vi "focusvi.vi"(1 "zc":dbl=5.0, 2 "yc":dbl, 3 "xc":dbl) -> (0 "finalz":dbl)   [LabVIEW 2015]
uses:
  <vilib>/Utility/miscctls.llb/LVOffsetAndMultiplierTypeDef.ctl
  <vilib>/DAQmx/read.llb/DAQmx Read (Analog 2D I16 NChan NSamp).vi
  <vilib>/DAQmx/write.llb/DAQmx Write (Analog DBL 1Chan 1Samp).vi
  Misc/add channel to active arrayv2.vi
  <vilib>/DAQmx/miscellaneous.llb/DAQmx Fill In Error Info.vi
  <vilib>/DAQmx/create/channels.llb/DAQmx Create Channel (AO-Voltage-Basic).vi
panel:
  in  "objective":u16(ring) items=["Olympus 25x NA 1.05", "Olympus 60x NA 1.2"]
  out "zsteps":i16
  out "ysteps":i16
  out "xsteps":i16
  out "samples":i32=18000
  in  "stop":bool
  in  "z-":bool
  in  "z+":bool
  in  "y+":bool
  in  "y-":bool
  in  "x+":bool
  in  "x-":bool
  in  "stepsize":dbl=0.005
  in  "zamp":dbl=0.25
  in  "y amp":dbl=0.25
  in  "x amp":dbl=0.25
  in  "samplingrate":dbl=18000.0
  in  "frametime (s)":dbl=1.0
  out "Waveform Graph 6":dbl[][](graph)=[[-0.004837577472790145, -0.005916214699391275, -0.005143459723331034, -0.0050629642879357565, -0.0055942334933206436, -0.004934171959757805, -0.004869775637052954, -0.005900115636177361, -0.004837577484431676, -0.005272252205759287, -0.00519175692461431, -0.005175657814834267, -0.004918072849977762, -0.005594233502051793, -0.0048214784445008265, -0.004563893371960148, -0.005191756977001205, -0.006286493106745184, -0.006318691279739141, -0.006431384710595012, -0.0047409831633558495, -0.00449949721514713, -0.005095162519137375, -0.005706926877610386, -0.005449341842904687, -0.004274110283586196, -0.004258011243655347, -0.00601280911359936, -0.005159558818559162, -0.004467299010138958, -0.005658629696699791, -0.005401044723112136, -0.0056425306131131945, -0.005465440975967795, -0.005030766304116696, -0.004499497218057513, -0.0048858746944461014, -0.004998568107839674, -0.005079063423909247, -0.005996709992177785, -0.004628289659740404, -0.0061416015611030165, -0.004531695364858024, -0.0050146671332186084, -0.005803521323832684, -0.005803521280176938, -0.004419001890346408, -0.005288351277704351, -0.0052078558917855846, -0.004354605649132282, -0.0052400540531380106, -0.004918072823784314, -0.006238195998594165, -0.004918072803411633, -0.004531695260084234, -0.006592375377658754, -0.005384945645346306, -0.003919930930715054, -0.003098878636956215, -0.005240054079331457, -0.0050790634355507795, -0.005223955085966736, -0.005513738165609539, -0.005578134371899068, -0.005417143856175244, -0.005143459711689502, -0.004274110251571983, -0.005352747463621199, -0.006705068866722286, -0.004402902800939046, -0.005626431608106941, -0.004982469088281505, -0.004934171901550144, -0.00588401664281264, -0.005368846619967371, -0.005787422135472298, -0.005143459743703715, -0.005449341842904687, -0.005884016584604979, -0.005626431573182345, -0.005513738165609539, -0.005690827895887196, -0.005449341936036944, -0.005497638962697238, -0.006205997802317143, -0.0052400540531380106, -0.004386803656234406, -0.00507906349375844, -0.005079063517041504, -0.005916214757598936, -0.005079063412267715, -0.0057391250040382145, -0.005916214716853574, -0.005143459673854522, -0.005755224090535194, -0.005610332533251494, -0.004354605588014237, -0.005417143751401454, -0.005384945636615157, -0.005352747425786219], [-0.004950270894914866, -0.005529837135691195, -0.004740983113879338, -0.004080921574495733, -0.0051595588098280135, -0.004644388775341212, -0.005175657826475799, -0.004612190602347255, -0.0058035212336108085, -0.005288351303897798, -0.00470878497872036, -0.006286493176594377, -0.0042741102486616, -0.004435100889531895, -0.005835719360038638, -0.00532054939540103, -0.005513738142326474, -0.005207855929620564, -0.003791138363885693, -0.00498246910283342, -0.00522395505104214, -0.0051112615590682255, -0.005401044804602862, -0.004805379404569976, -0.004982469041715376, -0.005159558771993034, -0.005401044629979879, -0.005175657838117331, -0.00546544095268473, -0.005352747399592772, -0.004982469032984227, -0.005143459662212991, -0.005240054125897587, -0.005578134371899068, -0.004934171889908611, -0.005465440987609327, -0.004966369981411844, -0.0050307662691921, -0.0041453178244410084, -0.004757082191645168, -0.005336648505181074, -0.004628289659740404, -0.0058035212336108085, -0.00618989875074476, -0.004740983081865125, -0.004918072800501249, -0.004901973728556186, -0.005159558771993034, -0.005288351280614734, -0.00522395505104214, -0.005674728751182556, -0.004869775645784102, -0.003952129045501351, -0.0045316952717257665, -0.0054171438212506475, -0.005175657791551202, -0.004918072780128568, -0.005240054085152224, -0.005352747533470393, -0.00561033247213345, -0.004934171820059419, -0.0056586296646855775, -0.005320549383759499, -0.005062964372336864, -0.005207855964545161, -0.005384945613332093, -0.00496636992902495, -0.0042902093147858976, -0.0045316953299334274, -0.005336648470256477, -0.004837577464058995, -0.00535274749272503, -0.005062964430544525, -0.005529837228823453, -0.005578134418465197, -0.004612190625630319, -0.006189898820593953, -0.004467299021780491, -0.004869775590486824, -0.00532054940413218, -0.005256153162918054, -0.004708784993272275, -0.004177515907213092, -0.004789280318072997, -0.004966370004694909, -0.005143459723331034, -0.006222096970304847, -0.005433242884464562, -0.005626431608106941, -0.005223954989924095, -0.004113119671819732, -0.004982469126116484, -0.005272252229042351, -0.004805379384197295, -0.004241912145516835, -0.005079063447192311, -0.0051595587545307355, -0.00607720531988889, -0.00578742225188762, -0.004419001864152961]]
  out "Waveform Graph 5":dbl[][](graph)=[[-0.005562035366892815, -0.005562035320326686, -0.005545936292037368, -0.005819620378315449, -0.0056103325448930265, -0.005256153139634989, -0.005384945645346306, -0.004998568102018907, -0.004676586796995253, -0.005288351254421286, -0.005159558821469545, -0.005272252214490436, -0.005771323142107576, -0.005079063400626182, -0.004821478459052742, -0.00429020928859245, -0.0053205494303256275, -0.005465441034175456, -0.005240054044406861, -0.005030766234267503, -0.005336648458614946, -0.004982469126116484, -0.005626431596465409, -0.005095162440557033, -0.005674728751182556, -0.0055137382121756675, -0.005642530621844344, -0.0052239549084333705, -0.00401652529835701, -0.005207855996559374, -0.005851818434894085, -0.0056747287744656205, -0.005384945683181286, -0.005384945633704774, -0.004950270976405591, -0.00524005409097299, -0.005803521230700426, -0.005642530729528516, -0.004628289642278105, -0.004982469091191888, -0.004644388746237382, -0.00541714378632605, -0.005159558742889203, -0.005062964395619929, -0.005352747580036521, -0.005706926932907664, -0.005706926889251918, -0.005578134465031326, -0.005159558786544949, -0.0063830875558778645, -0.004467299015959725, -0.005529837182257325, -0.006189898774027825, -0.00614160159311723, -0.004708785028196871, -0.0054171437659533694, -0.005127360642654821, -0.005449341901112348, -0.004676586936693638, -0.004805379334720783, -0.004789280347176827, -0.005030766254640185, -0.00562643154989928, -0.005578134360257536, -0.0042580112116411325, -0.004998568119481206, -0.005175657800282352, -0.005433242846629582, -0.004338506443309598, -0.0056264315120643, -0.004789280294789933, -0.004097020631888881, -0.005529837205540389, -0.004950270941480994, -0.0054815399926155806, -0.005658629618119448, -0.005079063400626182, -0.005481539922766387, -0.005481540027540177, -0.0055459362803958355, -0.005175657835206948, -0.005288351254421286, -0.005803521303460002, -0.005401044641621411, -0.006173799707903526, -0.005401044720201753, -0.00461219068383798, -0.005851818341761827, -0.004724884033203125, -0.005996710085310042, -0.005014667171053588, -0.005545936338603496, -0.005095162510406226, -0.00581962033174932, -0.004531695286277682, -0.004209713998716324, -0.0037106430681888014, -0.006640672439243644, -0.005690827872604132, -0.005867917533032596], [-0.00441900179721415, -0.00557813432533294, -0.005900115612894297, -0.00470878496998921, -0.005384945645346306, -0.005159558728337288, -0.006012809133972041, -0.0068821584107354285, -0.004740983151714317, -0.005272252194117755, -0.00482147850561887, -0.004370704677421599, -0.005320549383759499, -0.005046865352778695, -0.005578134360257536, -0.005336648420779966, -0.006173799722455442, -0.005851818574592471, -0.004885874659521505, -0.005272252194117755, -0.005706926769926212, -0.006077205296605825, -0.005175657823565416, -0.0045155962376156825, -0.004853676550555974, -0.005658629676327109, -0.0050307662691921, -0.005062964381068014, -0.00495027091819793, -0.004837577504804358, -0.005594233397278004, -0.005272252226131968, -0.005562035320326686, -0.005642530668410473, -0.0050307662226259705, -0.005578134430106729, -0.005240054125897587, -0.005723025975748896, -0.004837577472790145, -0.005111261626007035, -0.004853676570928655, -0.0049663699930533765, -0.006415285679395311, -0.005256153162918054, -0.005272252100985498, -0.006383087439462543, -0.005256153189111501, -0.0051112615590682255, -0.004982469067908823, -0.005207855961634778, -0.004129218746675179, -0.005143459650571458, -0.004676586863934062, -0.00429020939336624, -0.004531695257173851, -0.005095162522047758, -0.006383087509311736, -0.004789280344266444, -0.006061106291599572, -0.005384945729747415, -0.004612190619809553, -0.005352747486904263, -0.004821478453231975, -0.00514345970004797, -0.004596091527491808, -0.005433242802973836, -0.005900115691474639, -0.004547794346581213, -0.006045007181819528, -0.005320549453608691, -0.005240054079331457, -0.006994851885247044, -0.004757082182914018, -0.004435100973933004, -0.005030766280833631, -0.004467299068346619, -0.005111261631827802, -0.00509516254242044, -0.00519175682857167, -0.0050951625453308225, -0.0051112615037709475, -0.005223955027759075, -0.0058679175563156605, -0.004612190599436872, -0.0043385065859183666, -0.006045007123611867, -0.0049824689864180986, -0.005014667205978185, -0.005062964395619929, -0.00486977563414257, -0.004869775648694485, -0.005223954978282564, -0.005111261538695544, -0.004885874700266868, -0.004644388661836274, -0.005739125050604343, -0.005465440871194005, -0.0050951625453308225, -0.004789280297700316, -0.005803521335474215]]
  out "Waveform Graph 4":dbl[][](graph)=[[-0.005288351234048605, -0.0044351008458761495, -0.005417143774684519, -0.005771323153749108, -0.005465441042906605, -0.006061106370179914, -0.004853676515631377, -0.0053205493371933695, -0.005562035366892815, -0.005417143780505285, -0.006045007274951786, -0.005723025952465832, -0.006302592321299016, -0.004676586855202914, -0.005835719406604767, -0.005223955016117543, -0.004209713984164409, -0.0055459363735280934, -0.004805379442404956, -0.004757082171272487, -0.005513738142326474, -0.005175657838117331, -0.0049985682097030805, -0.005062964337412268, -0.0060772053897380825, -0.0053849456220632416, -0.004740983198280447, -0.004869775587576441, -0.005723025984480046, -0.005674728751182556, -0.004869775590486824, -0.005562035297043621, -0.004628289677202702, -0.004644388679298572, -0.0051595587166957555, -0.005111261538695544, -0.004966370036709122, -0.005401044664904475, -0.0060772053897380825, -0.005723025975748896, -0.005433242837898433, -0.005320549372117967, -0.004708784993272275, -0.005095162484212779, -0.004918072870350443, -0.005706926877610386, -0.004901973725645803, -0.004435100883711129, -0.004660487800720148, -0.005288351347553543, -0.005256153177469969, -0.004821478447411209, -0.004708784967078827, -0.005562035366892815, -0.004644388679298572, -0.005658629792742431, -0.004258011269848793, -0.00483757744950708, -0.0048375774989835914, -0.0049019737634807825, -0.004918072823784314, -0.005723025975748896, -0.0056425306713208554, -0.005095162460929714, -0.0051273606484755875, -0.005272252205759287, -0.004724884137976915, -0.006238195998594165, -0.004563893505837769, -0.0054815399926155806, -0.004692685857298784, -0.004354605625849217, -0.005256153113441542, -0.005127360657206736, -0.004869775599217974, -0.005030766266281716, -0.004837577469879761, -0.005207855976186693, -0.005642530624754727, -0.005368846608325839, -0.006431384687311947, -0.005835719371680171, -0.005191756851854734, -0.005304450355470181, -0.005079063444281928, -0.005723025929182768, -0.005272252182476222, -0.004950270915287547, -0.0050146670750109475, -0.005610332611831836, -0.00457999249920249, -0.004885874662431888, -0.005626431581913493, -0.005095162498764694, -0.005674728727899492, -0.004773181278142147, -0.005175657849758863, -0.005964511854108423, -0.005240054032765329, -0.006157700694166124], [-0.005433242849539966, -0.0056747287744656205, -0.005175657916697674, -0.005497639137320221, -0.005771323200315237, -0.00559423347003758, -0.004016525283805095, -0.00517565777990967, -0.005014667203067802, -0.005739124969113618, -0.005433242849539966, -0.004483398119919002, -0.003839435672853142, -0.004805379395838827, -0.004467299018870108, -0.0056908278609626, -0.005884016584604979, -0.00532054939540103, -0.004918072815053165, -0.005014667194336653, -0.004177515939227305, -0.005240054056048393, -0.005256153142545373, -0.0054654409410431985, -0.004934171913191676, -0.005368846585042775, -0.005095162484212779, -0.00538494570646435, -0.004225813108496368, -0.0050468652916606516, -0.0055781344417482615, -0.005159558771993034, -0.005401044664904475, -0.005207855952903628, -0.004515596255077981, -0.005288351257331669, -0.00536884656175971, -0.0049019737838534635, -0.004982469114474952, -0.005932313832454383, -0.004306308436207473, -0.00546544101962354, -0.0055620353319682184, -0.0050146671681432055, -0.005062964372336864, -0.004274110292317346, -0.004789280274417251, -0.005207855848129839, -0.0055459362803958355, -0.005368846535566263, -0.005513738165609539, -0.004402902800939046, -0.004563893331214786, -0.005030766266281716, -0.005803521303460002, -0.00424191213096492, -0.004354605634580367, -0.005256153142545373, -0.004467298983945512, -0.005191756831482053, -0.004467299068346619, -0.005288351234048605, -0.00536884656175971, -0.005175657858490013, -0.0053366483887657525, -0.005352747533470393, -0.0063830874627456066, -0.0049180727772181855, -0.005159558705054223, -0.0050790634355507795, -0.005320549369207584, -0.006833861174527556, -0.00552983716770541, -0.005497639055829495, -0.005449341854546219, -0.004789280306431465, -0.004885874685714953, -0.005916214699391275, -0.004708784958347678, -0.004692685880581848, -0.005642530659679323, -0.005626431584823876, -0.004644388728775084, -0.004821478432859294, -0.005674728684243746, -0.005513738200534135, -0.005658629781100899, -0.006125502567738294, -0.004821478424128145, -0.005223954981192947, -0.005207855952903628, -0.005706926807761192, -0.005240054114256054, -0.005594233423471451, -0.005143459653481841, -0.0054815400508232415, -0.0044029027776559815, -0.0049663699930533765, -0.0052078558946959674, -0.005884016596246511]]
  in  "bin":dbl=20.0
  out "Waveform Graph 3":dbl[][](graph)=[[-0.002712501134374179, -0.002406618936220184, -0.0023100245656678454, -0.0024871142755728214, -0.002245628336095251, -0.00256760960619431, -0.002020241448190063, -0.0024227179790614175, -0.0020202414161758497, -0.002937888045562431, -0.0023261236550752074, -0.0019397461233893409, -0.0022295292728813365, -0.0017787554766982793, -0.0025837086490355433, -0.0023100245569366963, -0.0023744208185235037, -0.0022295292321359737, -0.002310024542384781, -0.0022778264275984837, -0.002116835827473551, -0.0024227179877925665, -0.002213430209667422, -0.002535411441931501, -0.002438817048096098, -0.0022456283215433357, -0.002503213344607502, -0.0021651329938322307, -0.002986185168265365, -0.002020241433638148, -0.002454916134593077, -0.0025676095974631608, -0.0024388170219026505, -0.002664203947642818, -0.0023905198991997167, -0.002004142355872318, -0.0023744208097923546, -0.0026159067871049046, -0.0027929964679060506, -0.002487114261020906, -0.002454916128772311, -0.001875349847250618, -0.0026320058066630738, -0.002132934870314784, -0.0024066189216682687, -0.002342222718289122, -0.0019397461001062766, -0.0025354114535730333, -0.0026320058677811176, -0.0025354114593937995, -0.0021490339480806143, -0.002358321737847291, -0.0026320058357669042, -0.002358321781503037, -0.002454916134593077, -0.002310024536564015, -0.002132934870314784, -0.0025032133125932887, -0.0020846376719418913, -0.0026320057979319243, -0.002197331137722358, -0.0023100245336536316, -0.0021973310853354634, -0.0021329348586732523, -0.0024227179936133327, -0.00232612362888176, -0.002503213335876353, -0.0025032133038621397, -0.002326123652164824, -0.0025354114652145652, -0.002213430171832442, -0.002245628336095251, -0.0023905198933789505, -0.002213430221308954, -0.0020685386116383597, -0.0022778264770749956, -0.0026803030079463495, -0.0023905198991997167, -0.0023905198584543543, -0.0022939254675293343, -0.0025676095683593303, -0.0028734917839756237, -0.0021651329705491664, -0.0024066189245786516, -0.002358321732026525, -0.0024710152094485236, -0.002503213327145204, -0.002760798344388604, -0.002277826436329633, -0.002197331114439294, -0.0025515104876831173, -0.0024388170626480133, -0.0027768973843194543, -0.0020685385970864445, -0.0024871142726624385, -0.0026964020740706473, -0.002792996456264518, -0.0021168358100112526, -0.0022778264275984837, -0.002374420821433887], [-0.0024227180139860137, -0.0023744207981508227, -0.002519312399090268, -0.0023422226775437595, -0.002229529243777506, -0.002567609556717798, -0.0024549160996684806, -0.0022617273643845692, -0.0022134301980258897, -0.0021973311435431243, -0.002213430157280527, -0.002471015212358907, -0.0022939254791708662, -0.002406618944951333, -0.002535411424469203, -0.002310024548205547, -0.0023905198584543543, -0.002116835824563168, -0.002438817039364949, -0.0025515105167869478, -0.0021007367526181043, -0.0025032133009517564, -0.002229529243777506, -0.0027768973930506037, -0.002728600206319243, -0.002471015203627758, -0.001939746068092063, -0.0024066189827863125, -0.002116835824563168, -0.001955845145857893, -0.0023100245656678454, -0.002165133022936061, -0.0027125011867610736, -0.0026481049018912016, -0.0021490339160664005, -0.0027446992986369877, -0.002503213330055587, -0.0025032133155036716, -0.0021651329909218473, -0.002326123625971377, -0.002068538617459126, -0.0023422226717229933, -0.0027607983152847736, -0.0024710151774343103, -0.0022134301863843573, -0.0022134301892947406, -0.0018270526605192571, -0.002744699252070859, -0.0025032133125932887, -0.0026320058037526905, -0.002471015212358907, -0.0021651329851010816, -0.0026320058124838395, -0.0023261236026883127, -0.0025998076889663935, -0.0025837086082901805, -0.0020363404968520627, -0.002664204002940096, -0.002245628274977207, -0.0025354114535730333, -0.0023583217873238025, -0.002068538608727977, -0.0025354114768560976, -0.002277826424688101, -0.0024549161695176735, -0.0021490339393494652, -0.0025515104993246497, -0.002052439551334828, -0.0021007367438869553, -0.0022134301892947406, -0.0023583217291161416, -0.002873491813079454, -0.0020041423529619353, -0.0024227180139860137, -0.002197331137722358, -0.0023100245802197606, -0.0029700861865421756, -0.0024549161025788635, -0.0024549161695176735, -0.0017948545544641092, -0.0027768974483478813, -0.0022617273381911216, -0.0024710151861654594, -0.0027768973930506037, -0.001988043324672617, -0.0024710151978069917, -0.0024388170917518438, -0.002245628341916017, -0.0022617273789364845, -0.0019236470601754264, -0.0026642039709258826, -0.0026320058357669042, -0.0026803030661540104, -0.0024710152443731203, -0.002632005824125372, -0.0023583217611303554, -0.0018914489191956818, -0.0023905198584543543, -0.0021651329938322307, -0.002374420812702738]]
  out "Waveform Graph 2":dbl[][](graph)=[[-0.0022939254879020153, -0.0025676095916423946, -0.002132934902328998, -0.002374420821433887, -0.002390519852633588, -0.002277826436329633, -0.002036340444465168, -0.0026964020653394982, -0.0024388171033933757, -0.0027286002004984766, -0.002374420838896185, -0.002712501146015711, -0.0021812320541357622, -0.002245628318632953, -0.0022939254500670358, -0.0022617273789364845, -0.002583708643214777, -0.002020241413265467, -0.0024710151890758427, -0.002567609547986649, -0.002100736740976572, -0.0024871142988558857, -0.002197331073693931, -0.0025032132922206073, -0.00258370864612516, -0.0021329348644940184, -0.0024710151861654594, -0.002084637639927678, -0.0029861852177418768, -0.0022617273876676335, -0.0025193124020006508, -0.002100736749707721, -0.0024871142813935876, -0.0026481049018912016, -0.002132934870314784, -0.0024388170888414605, -0.002712501198402606, -0.0018592507723951713, -0.0028251945797819642, -0.0022456283011706548, -0.002326123634702526, -0.0022939255024539305, -0.0022456282924395053, -0.002615906766732223, -0.0028734917956171556, -0.002342222651350312, -0.0022295292641501875, -0.0023100245773093773, -0.00255151052842848, -0.002132934870314784, -0.002326123637612909, -0.0019397461146581918, -0.002068538626190275, -0.00263200584158767, -0.00250321333296597, -0.0025837086228420957, -0.001843151735374704, -0.002551510540070012, -0.0026642039738362655, -0.0022134301834739745, -0.002760798318195157, -0.0024227179877925665, -0.0022134301892947406, -0.002454916131682694, -0.0021168358158320188, -0.0023261236143298446, -0.0022939254675293343, -0.0029056899016723036, -0.002149033942259848, -0.0022778264508815484, -0.002776897407602519, -0.0022295292699709536, -0.002970086151617579, -0.0023905198817374186, -0.002052439545514062, -0.002406618936220184, -0.0020685385970864445, -0.0024388170626480133, -0.002261727346922271, -0.0022456283128121867, -0.0020685385999968274, -0.0024066189653240144, -0.0028573927120305598, -0.002406618944951333, -0.0020685386029072107, -0.0020846376894041894, -0.0026159067638218403, -0.0025676095974631608, -0.0021973311493638905, -0.00243881705973763, -0.002277826456702314, -0.0023583217611303554, -0.0025032133475178854, -0.0021812320599565284, -0.002422717970330268, -0.002326123617240228, -0.0024227180372690784, -0.00253541145066265, -0.002197331123170443, -0.002277826430508867], [-0.0030183833790943027, -0.0022778264625230803, -0.0021973310998873786, -0.002213430195115507, -0.002245628327364102, -0.0027607983094640074, -0.0022134301834739745, -0.002438817048096098, -0.002358321749488823, -0.002599807700607926, -0.0023422226833645253, -0.0020041423675138505, -0.002310024562757462, -0.002229529246687889, -0.0020846376690315084, -0.002149033918976784, -0.00232612362888176, -0.0023744208097923546, -0.0022456282895291224, -0.0024066189740551635, -0.0027768973843194543, -0.0023583217873238025, -0.0025998076802352444, -0.0017304582783253864, -0.0025354114623041824, -0.0021812320774188265, -0.002293925514095463, -0.002728600238333456, -0.002310024594771676, -0.0026481048815185206, -0.0025354114186484367, -0.0023261236638063565, -0.002889590832637623, -0.0019719442148925736, -0.002648104846593924, -0.0022939254966331648, -0.0021007367584388705, -0.0023100245685782283, -0.0018592507723951713, -0.002229529261239804, -0.001794854539912194, -0.002100736732245423, -0.0022456283011706548, -0.0020363404997624456, -0.0023100245598470792, -0.0023744208505377174, -0.0022295292641501875, -0.002197331128991209, -0.0029378880222793668, -0.0024227179819718003, -0.0021812320599565284, -0.002615906758001074, -0.002020241430727765, -0.00245491613750346, -0.0022617273643845692, -0.0026159067725529893, -0.002535411424469203, -0.0021168358158320188, -0.002535411456483416, -0.0022617273876676335, -0.0021651330025633797, -0.002503213330055587, -0.0026159067725529893, -0.002873491760692559, -0.0021007367206038905, -0.002632005856139585, -0.002229529229225591, -0.0024388170859310776, -0.0023261236114194618, -0.002454916134593077, -0.002277826430508867, -0.0026803030603332447, -0.0025032133155036716, -0.002116835772176273, -0.002390519896289334, -0.002261727358563803, -0.002277826436329633, -0.0024871142726624385, -0.0023905198933789505, -0.001971944238175638, -0.002825194620527327, -0.0019558451895136386, -0.002583708660677075, -0.002615906746359542, -0.002358321737847291, -0.0024227180023444817, -0.002326123640523292, -0.0026481048844289035, -0.0023100245685782283, -0.0024871142493793743, -0.0018753498385194688, -0.0022617273760261016, -0.0028573927644174545, -0.0020685385941760616, -0.002326123643433675, -0.0023100245598470792, -0.002358321743668057, -0.002664203947642818, -0.0021651330025633797, -0.0025193123874487355]]
  out "Waveform Graph":dbl[][](graph)=[[-0.0021168357983697207, -0.0025837086694082247, -0.002438817106303759, -0.0024066189595032482, -0.002712501122732647, -0.002004142350051552, -0.002728600229602307, -0.0024066189565928654, -0.002503213324234821, -0.0020846377010457218, -0.002052439551334828, -0.002454916114220396, -0.002599807741353288, -0.002004142408259213, -0.002358321743668057, -0.0022778264508815484, -0.0025354114535730333, -0.0025676095770904793, -0.002519312355434522, -0.0022456282895291224, -0.0025354114652145652, -0.0025354114535730333, -0.002277826424688101, -0.0024066189565928654, -0.002358321755309589, -0.001971944217802957, -0.002953987114597112, -0.00243881705973763, -0.0021490339218871667, -0.002551510473131202, -0.0021007367642596362, -0.0030505814647767693, -0.0022456283128121867, -0.00232612362888176, -0.0021651329909218473, -0.002825194603065029, -0.0025193123932695017, -0.0023422226920956747, -0.0025032133533386515, -0.0021490339306183158, -0.0022939254733501, -0.0028251946088857947, -0.0022778264537919313, -0.0027286001946777104, -0.002020241427817382, -0.002293925525736995, -0.002744699286995456, -0.002471015229821205, -0.0024388170830206947, -0.002084637666121125, -0.002664204002940096, -0.0024388170888414605, -0.0024066189886070787, -0.002181232051225379, -0.0021812320774188265, -0.0025193123816279694, -0.0023100245802197606, -0.0019075479824095965, -0.0028090955194784327, -0.0021168358100112526, -0.0026320058532292023, -0.002680303025408648, -0.002454916149144992, -0.0024227179994340984, -0.002422718011075631, -0.0022778264450607822, -0.00276079832110554, -0.002374420789419673, -0.00243881705973763, -0.002277826430508867, -0.0024710151978069917, -0.002374420812702738, -0.002358321743668057, -0.002422718022717163, -0.002036340479389764, -0.002728600226691924, -0.002052439554245211, -0.002551510505145416, -0.0020363404852105304, -0.002293925525736995, -0.0023583217291161416, -0.002374420835985802, -0.0024388170830206947, -0.002100736746797338, -0.0022134301834739745, -0.002567609545076266, -0.0025837086577666923, -0.0024227179994340984, -0.002181232045404613, -0.0020846376719418913, -0.0027125011751195417, -0.0021168358071008697, -0.0028412936633685605, -0.0021007367526181043, -0.0022778264596126974, -0.00253541145066265, -0.0025193123903591184, -0.0021007367438869553, -0.002197331137722358, -0.002471015159972012], [-0.002293925522826612, -0.00224562827788759, -0.002358321743668057, -0.002390519846812822, -0.002149033936439082, -0.0019397461030166597, -0.002841293692472391, -0.0022939254908123986, -0.002422718008165248, -0.0022295292728813365, -0.002342222718289122, -0.0030988786573288964, -0.0022939255082746967, -0.002052439545514062, -0.0020363404561067, -0.0025676095800008627, -0.0027929964679060506, -0.0023583217262057588, -0.0024871143163181842, -0.0019558451720513405, -0.0025676095916423946, -0.0024066189595032482, -0.002310024548205547, -0.0025032133649801835, -0.0020041423733346162, -0.0023100245656678454, -0.0023905198875581847, -0.002261727390578017, -0.002615906743449159, -0.0019880432984791694, -0.00245491613750346, -0.002535411430289969, -0.002004142355872318, -0.0023422226920956747, -0.00243881705973763, -0.002632005832856521, -0.002245628318632953, -0.0022778264275984837, -0.0018753498676232993, -0.002197331114439294, -0.0022939254937227815, -0.002132934852852486, -0.0023583217640407383, -0.002744699301547371, -0.002471015203627758, -0.0030183833732735366, -0.0026320058706915004, -0.002229529246687889, -0.002358321723295376, -0.0025998077064286916, -0.0024549161578761415, -0.0021812320221215485, -0.002406618933309801, -0.0019397460971958935, -0.0027607982978224755, -0.002358321743668057, -0.002342222660081461, -0.0026642039243597536, -0.0022456282953498886, -0.0027929964620852844, -0.00231002455111593, -0.002454916134593077, -0.0024066189478617163, -0.0018431517150020228, -0.003066680557094514, -0.002471015203627758, -0.002599807741353288, -0.00243881705973763, -0.0023261236026883127, -0.0024549161607865244, -0.0024871142668416724, -0.002406618936220184, -0.0021973311027977615, -0.0018109535943949596, -0.003066680516349152, -0.002454916149144992, -0.00231002455111593, -0.002245628333184868, -0.0025515105342492463, -0.00247101521526929, -0.002293925514095463, -0.002712501137284562, -0.0022617273760261016, -0.002535411447752267, -0.0025032133562490344, -0.0019719442236237226, -0.0023744207923300565, -0.00195584520988632, -0.0024227179936133327, -0.0025998076860560106, -0.002422718022717163, -0.002680303010856733, -0.002229529246687889, -0.0024066189565928654, -0.0023583217669511216, -0.002583708643214777, -0.002197331123170443, -0.001988043283927254, -0.002454916149144992, -0.002583708634483628]]
  # "X"
  # "Y"
  # "Z"
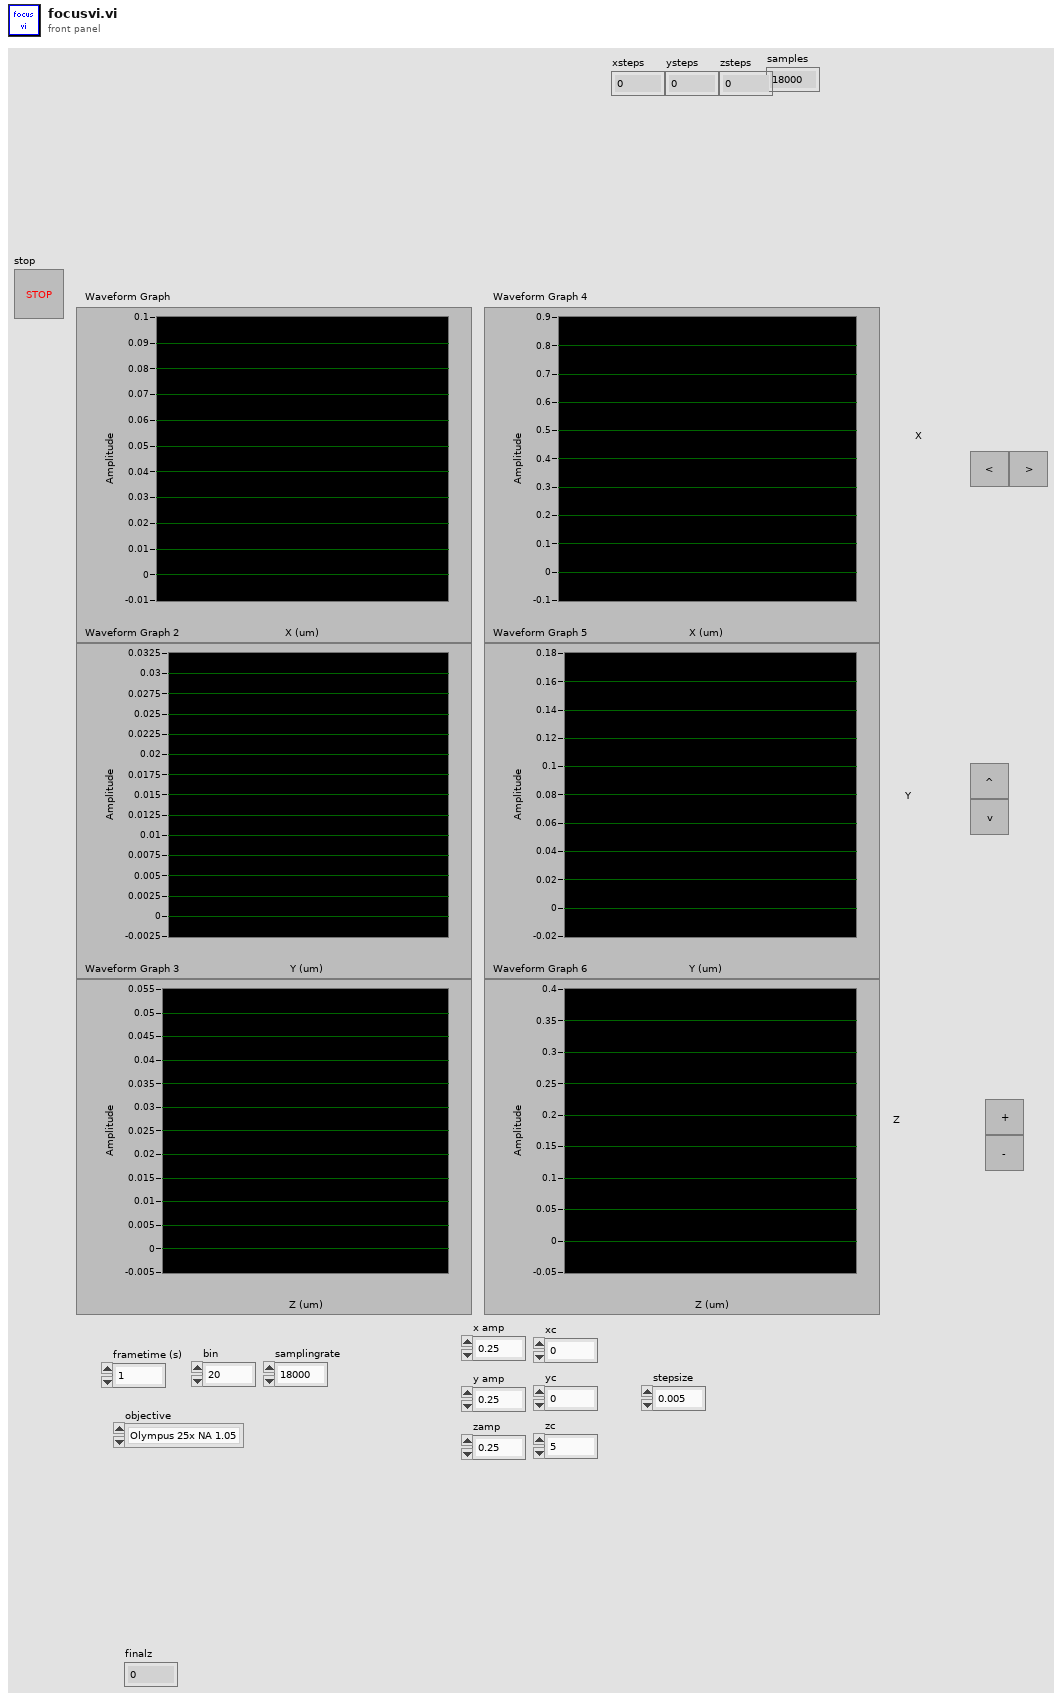
[diagram p1: front panel]
types:
  T1 = typedef "LVOffsetAndMultiplierTypeDef.ctl" = cluster{"Offset":dbl, "Multiplier":dbl}
  T2 = cluster{"presorted indices":i32[], "AOchans in this device":tag[], "usedAO sorted":i32[]}[]
  T3 = cluster{"StageS":i32, "StageL":i32, "currmeas data dir":path, "image OD":u16, "contour OD":u16, "point OD":u16, "AOlines":tag[], "AIlines":tag[], "CI lines":tag[], "DO lines":tag[], "AO names":string[], "CI names":string[], "AI names":string[], "DO names":string[], "CIextensions":string[], "AIextensions":string[], "Voltage to Ygalvo":i32, "Voltage to Xgalvo":i32, "Voltage to patch":i32, "640 shutter":i32, "2P shutter":i32, "LT timestamp":u32, "Vp":i32, "Ip":i32, "camera trigger":i32, "master data dir":path, "voltage to Zpos":i32, "Vto2P":i32, "640 AO":i32, "488 AO":i32, "532 AO":i32, "640TTL":u32, "488TTL":u32, "532TTL":u32, "Device 1 sampleclock out":tag, "Device 1 Starttrigger out":tag, "Device 2 sampleclock in":tag, "Device 2 StartTrigger in ":tag, "2PODTTL":u32, "488 shutter":u32, "LCVR red":u32, "LCVR blue":u32}
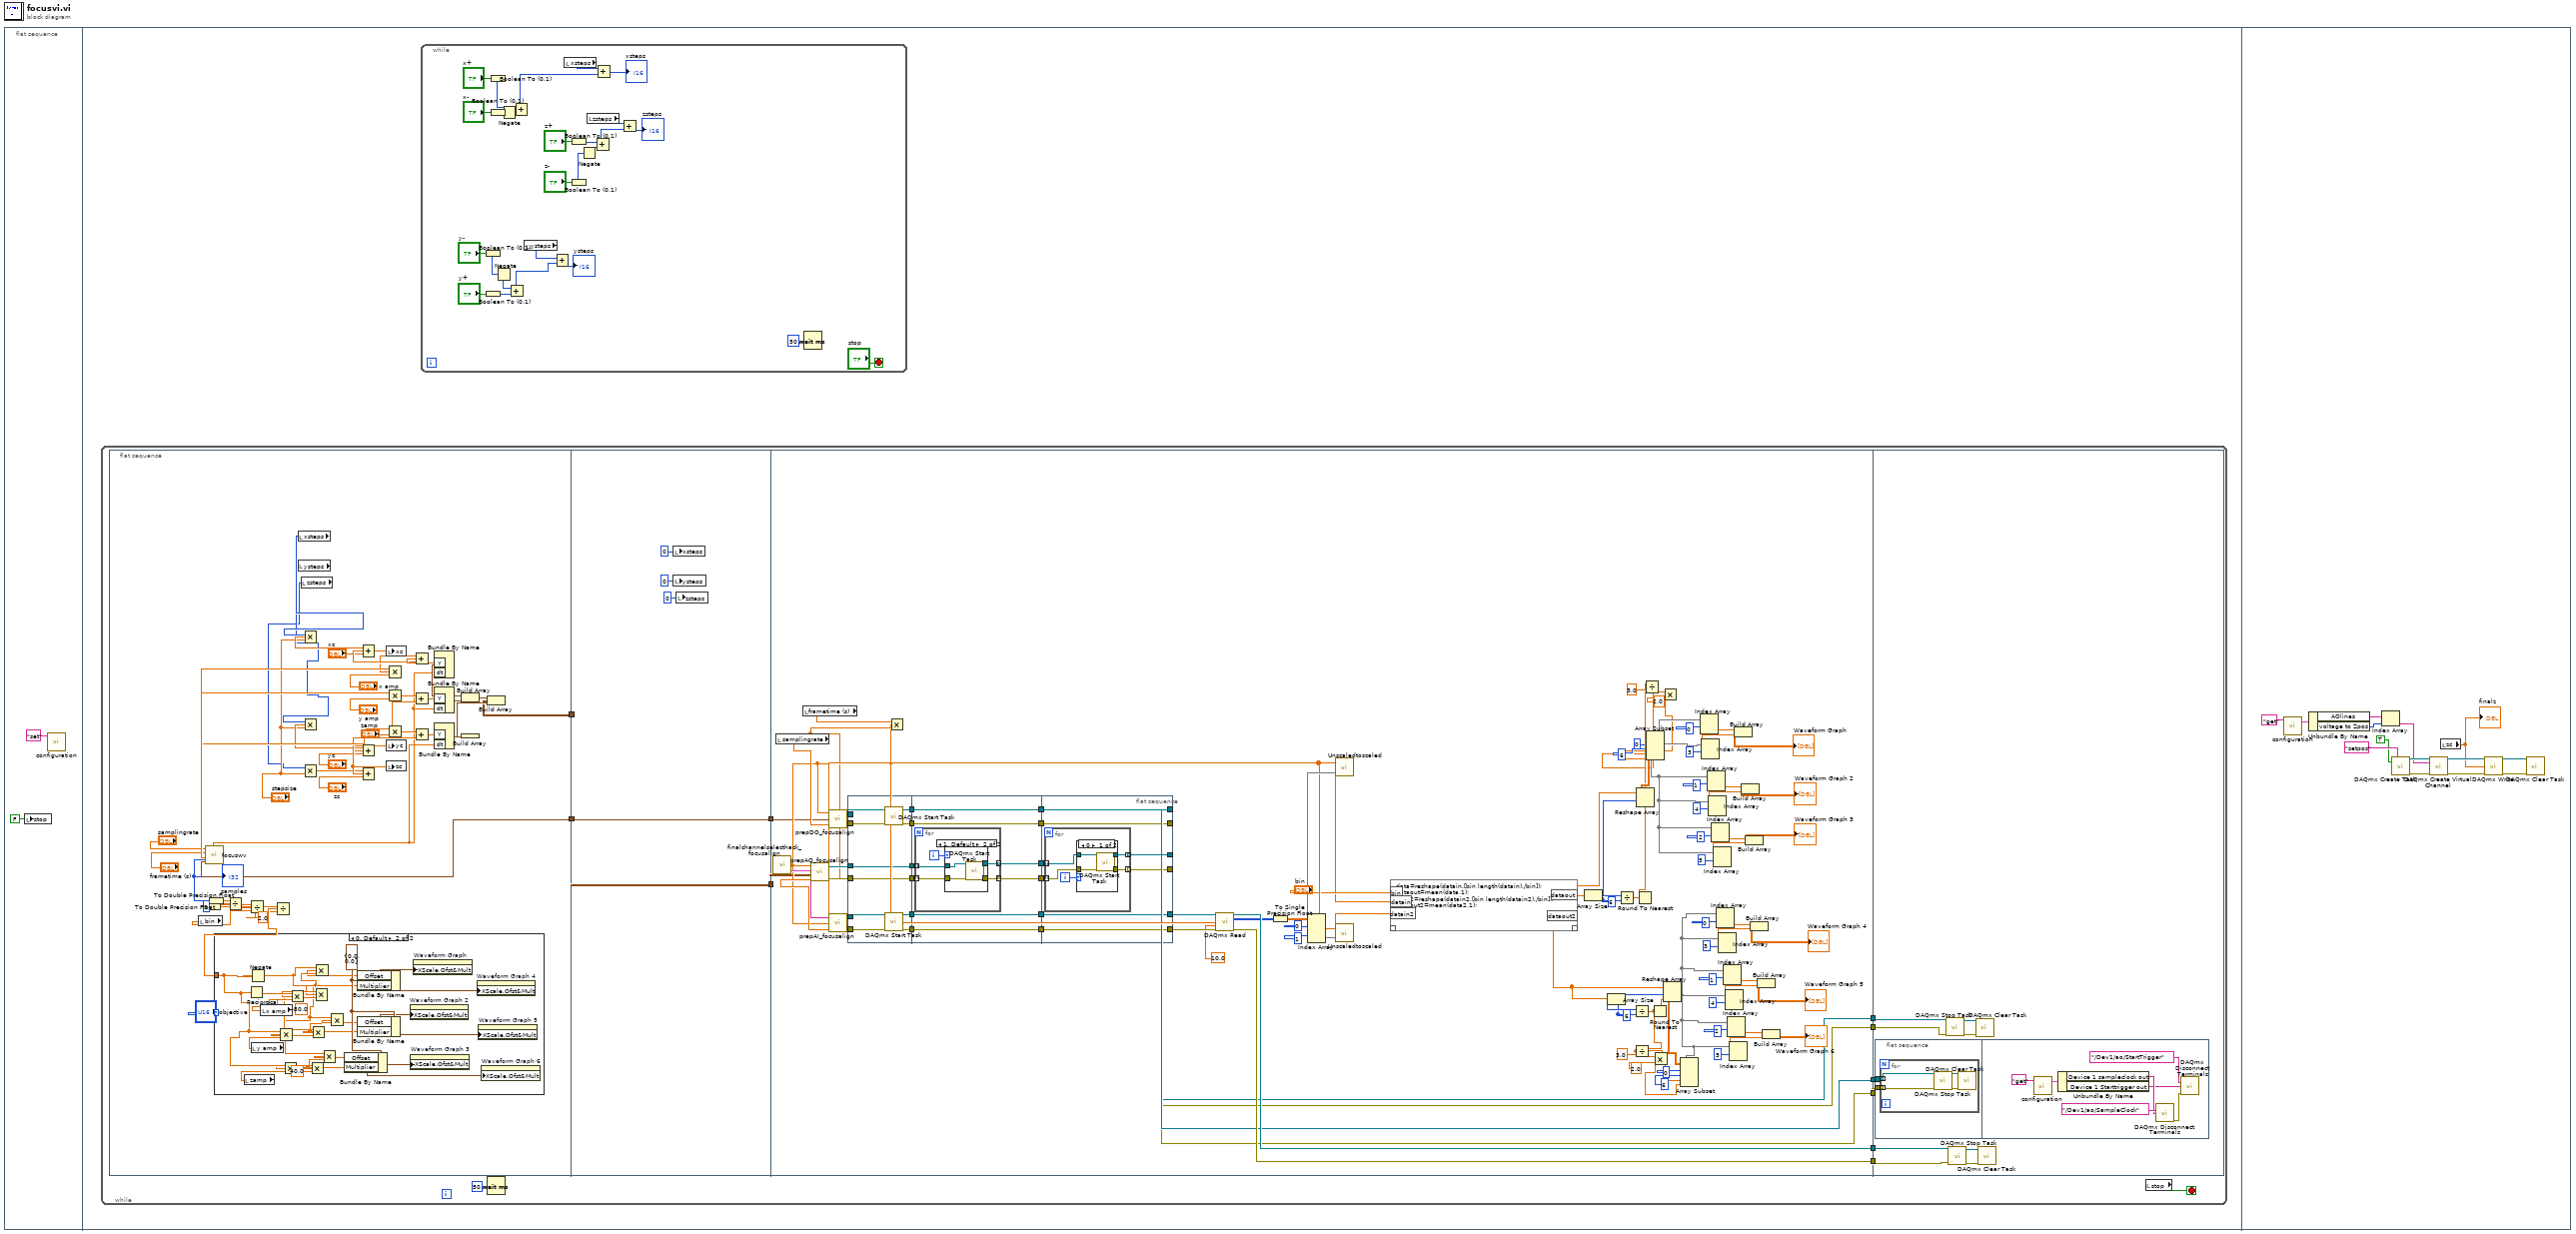
[diagram p0: block diagram]
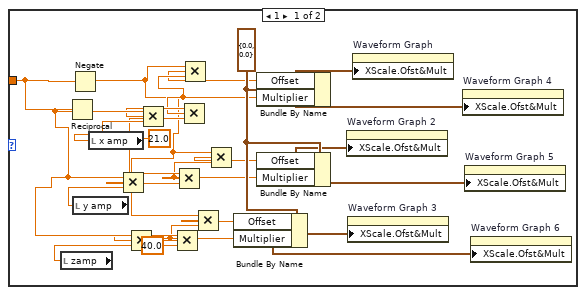
[diagram p2: hidden frame]
diagram:
  n1 = flat-sequence {
    frame #0 {
      n2 = local write "stop"(FALSE ("stop")) -> ()
      n3 = call "configuration.vi"("command"="set") -> ()  [unwired: 2 in, 2 out]
    }
    frame #1 {
      n4 = while {
        stop <- w14 stop-if-true
        n5 = flat-sequence {
          tunnel: [w26] -> w5
          tunnel: [w25] -> w3
          tunnel: [w103] -> w6
          tunnel: w5 -> [w103]
          tunnel: [w102] -> w4
          tunnel: w3 -> [w102]
          tunnel: [w134] -> w13
          tunnel: [w133] -> w12
          tunnel: [w132] -> w11
          tunnel: [w131] -> w10
          tunnel: [w130] -> w9
          tunnel: [w129] -> w8
          tunnel: w6 -> [w128]
          tunnel: w4 -> [w127]
          tunnel: w13 -> [w260]
          tunnel: w12 -> [w259]
          tunnel: w11 -> [w258]
          tunnel: w10 -> [w257]
          tunnel: w9 -> [w256]
          tunnel: w8 -> [w255]
          frame #0 {
            n6 = local read "bin"() -> (w18:dbl)
            n7 = To Double Precision Float(number=9 ("y")) -> (double precision float=w20:dbl)
            n8 = call "focuswv.vi"("frametime (s)"="frametime (s)", "samplingrate"="samplingrate") -> ("digwfs"=w25:digitalwaveform[], "YV"=w56:dbl[], "ZV"=w54:dbl[], "XV"=w55:dbl[], "samples"=w23:i32, "dt"=w38:dbl)  [unwired: 2 in]
            "samples" <- w23
            n9 = To Double Precision Float(number=w23) -> (double precision float=w21:dbl)
            n10 = Divide(x=w21, y=w20) -> (x/y=w19:dbl)
            n11 = Divide(x=w19, y=w18) -> (x/y=w17:dbl)
            n12 = Divide(x=w17, y=2.0) -> (x/y=w16:dbl)
            n13 = case shown="0, Default" "objective" {
              tunnel: w16 -> [w80 w101]
              frame 1 {
                w69 = T1 {"Offset"=0.0, "Multiplier"=0.0} ("X Scale.Offset and Multiplier")
                w74 = 21.0 ("y")
                n14 = local read "zamp"() -> (w78:dbl)
                n15 = Reciprocal(x=w80) -> (1/x=w77:dbl)
                n16 = Negate(x=w80) -> (-x=w60:dbl)
                n17 = local read "y amp"() -> (w76:dbl)
                n18 = local read "x amp"() -> (w79:dbl)
                n19 = Multiply(x=w77, y=w76) -> (x*y=w73:dbl)
                n20 = Multiply(x=w77, y=w78) -> (x*y=w72:dbl)
                n21 = Multiply(x=w77, y=w79) -> (x*y=w75:dbl)
                n22 = Multiply(x=w72, y=40.0) -> (x*y=w62:dbl)
                n23 = Multiply(x=w74, y=w73) -> (x*y=w63:dbl)
                n24 = Multiply(x=w75, y=w74) -> (x*y=w66:dbl)
                n25 = Multiply(x=w60, y=w66) -> (x*y=w65:dbl)
                n26 = Multiply(x=w60, y=w62) -> (x*y=w61:dbl)
                n27 = Multiply(x=w60, y=w63) -> (x*y=w64:dbl)
                n28 = Bundle By Name(cluster=w69, "Offset"=w61, "Multiplier"=w62) -> (w67:T1)
                n29 = Bundle By Name(cluster=w69, "Offset"=w65, "Multiplier"=w66) -> (w70:T1)
                n30 = Bundle By Name(cluster=w69, "Offset"=w64, "Multiplier"=w63) -> (w68:T1)
                n31 = property on="Waveform Graph 2" class="WFGraph (strict)"("XScale.Ofst&Mult"=w68) -> ()  [unwired: 2 in, 2 out]
                n32 = property on="Waveform Graph 3" class="WFGraph (strict)"("XScale.Ofst&Mult"=w67) -> ()  [unwired: 2 in, 2 out]
                n33 = property on="Waveform Graph" class="WFGraph (strict)"("XScale.Ofst&Mult"=w70) -> ()  [unwired: 2 in, 2 out]
                n34 = property on="Waveform Graph 4" class="WFGraph (strict)"("XScale.Ofst&Mult"=w70) -> ()  [unwired: 2 in, 2 out]
                n35 = property on="Waveform Graph 5" class="WFGraph (strict)"("XScale.Ofst&Mult"=w68) -> ()  [unwired: 2 in, 2 out]
                n36 = property on="Waveform Graph 6" class="WFGraph (strict)"("XScale.Ofst&Mult"=w67) -> ()  [unwired: 2 in, 2 out]
              }
              frame 0, Default {
                w90 = T1 {"Offset"=0.0, "Multiplier"=0.0} ("X Scale.Offset and Multiplier")
                w95 = 50.0 ("y")
                n37 = local read "zamp"() -> (w99:dbl)
                n38 = Reciprocal(x=w101) -> (1/x=w98:dbl)
                n39 = Negate(x=w101) -> (-x=w81:dbl)
                n40 = local read "y amp"() -> (w97:dbl)
                n41 = local read "x amp"() -> (w100:dbl)
                n42 = Multiply(x=w98, y=w97) -> (x*y=w94:dbl)
                n43 = Multiply(x=w98, y=w99) -> (x*y=w93:dbl)
                n44 = Multiply(x=w98, y=w100) -> (x*y=w96:dbl)
                n45 = Multiply(x=w93, y=40.0) -> (x*y=w83:dbl)
                n46 = Multiply(x=w95, y=w94) -> (x*y=w84:dbl)
                n47 = Multiply(x=w96, y=w95) -> (x*y=w87:dbl)
                n48 = Multiply(x=w81, y=w87) -> (x*y=w86:dbl)
                n49 = Multiply(x=w81, y=w83) -> (x*y=w82:dbl)
                n50 = Multiply(x=w81, y=w84) -> (x*y=w85:dbl)
                n51 = Bundle By Name(cluster=w90, "Offset"=w82, "Multiplier"=w83) -> (w88:T1)
                n52 = Bundle By Name(cluster=w90, "Offset"=w86, "Multiplier"=w87) -> (w91:T1)
                n53 = Bundle By Name(cluster=w90, "Offset"=w85, "Multiplier"=w84) -> (w89:T1)
                n54 = property on="Waveform Graph 2" class="WFGraph (strict)"("XScale.Ofst&Mult"=w89) -> ()  [unwired: 2 in, 2 out]
                n55 = property on="Waveform Graph 3" class="WFGraph (strict)"("XScale.Ofst&Mult"=w88) -> ()  [unwired: 2 in, 2 out]
                n56 = property on="Waveform Graph" class="WFGraph (strict)"("XScale.Ofst&Mult"=w91) -> ()  [unwired: 2 in, 2 out]
                n57 = property on="Waveform Graph 4" class="WFGraph (strict)"("XScale.Ofst&Mult"=w91) -> ()  [unwired: 2 in, 2 out]
                n58 = property on="Waveform Graph 5" class="WFGraph (strict)"("XScale.Ofst&Mult"=w89) -> ()  [unwired: 2 in, 2 out]
                n59 = property on="Waveform Graph 6" class="WFGraph (strict)"("XScale.Ofst&Mult"=w88) -> ()  [unwired: 2 in, 2 out]
              }
            }
            n60 = local read "xsteps"() -> (w29:i16)
            n61 = local read "ysteps"() -> (w28:i16)
            n62 = local read "zsteps"() -> (w27:i16)
            n63 = Multiply(x=w29, y="stepsize") -> (x*y=w31:dbl)
            n64 = Multiply(x=w28, y="stepsize") -> (x*y=w32:dbl)
            n65 = Multiply(x=w27, y="stepsize") -> (x*y=w33:dbl)
            n66 = Add(x=w31, y="xc") -> (x+y=w45:dbl)
            n67 = Add(x=w32, y="yc") -> (x+y=w46:dbl)
            n68 = Add(x=w33, y="zc") -> (x+y=w47:dbl)
            n69 = local write "xc"(w45) -> ()
            n70 = Multiply(x=w55, y="x amp") -> (x*y=w42:dbl[])
            n71 = Multiply(x=w56, y="y amp") -> (x*y=w43:dbl[])
            n72 = Multiply(x=w54, y="zamp") -> (x*y=w44:dbl[])
            n73 = local write "yc"(w46) -> ()
            n74 = local write "zc"(w47) -> ()
            n75 = Add(x=w42, y=w45) -> (x+y=w57:dbl[])
            n76 = Add(x=w43, y=w46) -> (x+y=w58:dbl[])
            n77 = Add(x=w44, y=w47) -> (x+y=w59:dbl[])
            n78 = Bundle By Name("Y"=w57, "dt"=w38) -> (w49:waveform(dbl))  [unwired: 1 in]
            n79 = Bundle By Name("Y"=w58, "dt"=w38) -> (w48:waveform(dbl))  [unwired: 1 in]
            n80 = Bundle By Name("Y"=w59, "dt"=w38) -> (w50:waveform(dbl))  [unwired: 1 in]
            n81 = Build Array(w49, w48) -> (w51:waveform(dbl)[])
            n82 = Build Array(w50) -> (w52:waveform(dbl)[])
            n83 = Build Array(w51, w52) -> (w26:waveform(dbl)[][])
          }
          frame #1 {
            n84 = local write "xsteps"(i16 0 ("xsteps")) -> ()
            n85 = local write "ysteps"(i16 0 ("ysteps")) -> ()
            n86 = local write "zsteps"(i16 0 ("zsteps")) -> ()
          }
          frame #2 {
            w120 = 6 ("y")
            w117 = 6 ("y")
            n87 = call "finalchannelselecthack_focusalign.vi"() -> ("Device chans"=w194:T2)  [unwired: 1 in, 1 out]
            n88 = local read "samplingrate"() -> (w137:dbl)
            n89 = local read "frametime (s)"() -> (w138:dbl)
            n90 = flat-sequence {
              tunnel: w191 -> [w215]
              tunnel: w192 -> [w216]
              tunnel: [w216] -> w206
              tunnel: [w215] -> w205
              tunnel: w190 -> [w214]
              tunnel: w189 -> [w213]
              tunnel: [w212] -> w204
              tunnel: [w211] -> w203
              tunnel: w188 -> [w210]
              tunnel: w187 -> [w209]
              tunnel: [w208] -> w202
              tunnel: [w207] -> w201
              tunnel: [w222] -> w200
              tunnel: [w221] -> w199
              tunnel: w206 -> [w224]
              tunnel: w205 -> [w223]
              tunnel: [w220] -> w198
              tunnel: w204 -> [w220]
              tunnel: [w219] -> w197
              tunnel: w203 -> [w219]
              tunnel: [w218] -> w196
              tunnel: w202 -> [w218]
              tunnel: [w217] -> w195
              tunnel: w201 -> [w217]
              tunnel: w200 -> [w243]
              tunnel: w199 -> [w242]
              tunnel: [w241] -> w132
              tunnel: [w240] -> w131
              tunnel: [w239] -> w186
              tunnel: w198 -> [w239]
              tunnel: [w238] -> w185
              tunnel: w197 -> [w238]
              tunnel: [w237] -> w130
              tunnel: w196 -> [w237]
              tunnel: [w236] -> w129
              tunnel: w195 -> [w236]
              frame #0 {
                n91 = call <vilib>:"DAQmx Start Task.vi"("task/channels in"=w210, "error in"=w209) -> ("task out"=w208:refnum<k21>, "error out"=w207:errorcluster)  [unwired: 12 in]
                n92 = call <vilib>:"DAQmx Start Task.vi"("task/channels in"=w214, "error in"=w213) -> ("task out"=w212:refnum<k21>, "error out"=w211:errorcluster)  [unwired: 12 in]
              }
              frame #1 {
                n93 = for {
                  tunnel: w224 -> [w229] mode=indexing
                  tunnel: [w226] -> w221 mode=indexing
                  tunnel: w223 -> [w227] mode=indexing
                  tunnel: [w228] -> w222 mode=indexing
                  i -> [w225]
                  n94 = case shown="1, Default" w225 {
                    tunnel: w229 -> [w231 w235]
                    tunnel: [w231 w234] -> w228
                    tunnel: w227 -> [w230 w233]
                    tunnel: [w230 w232] -> w226
                    frame 0 {
                    }
                    frame 1, Default {
                      n95 = call <vilib>:"DAQmx Start Task.vi"("task/channels in"=w235, "error in"=w233) -> ("task out"=w234:refnum<k21>, "error out"=w232:errorcluster)  [unwired: 12 in]
                    }
                  }
                }
              }
              frame #2 {
                n96 = for {
                  tunnel: w243 -> [w248] mode=indexing
                  tunnel: w242 -> [w247] mode=indexing
                  tunnel: [w246] -> w241 mode=indexing
                  tunnel: [w245] -> w240 mode=indexing
                  i -> [w244]
                  n97 = case shown="0" w244 {
                    tunnel: w248 -> [w252 w253]
                    tunnel: w247 -> [w251 w254]
                    tunnel: [w250 w253] -> w246
                    tunnel: [w249 w254] -> w245
                    frame 0 {
                      n98 = call <vilib>:"DAQmx Start Task.vi"("task/channels in"=w252, "error in"=w251) -> ("task out"=w250:refnum<k21>, "error out"=w249:errorcluster)  [unwired: 12 in]
                    }
                    frame 1, Default {
                    }
                  }
                }
              }
            }
            n99 = Multiply(x=w138, y=w137) -> (x*y=w136:dbl)
            n100 = call "prepAO_focusalign.vi"("srate"=w137, "waveforms"=w128, "Device chans"=w194, "bufferAO"=w136) -> ("AOerrout"=w191:errorcluster[], "Terminal Name with Device Prefix"=w193:tag, "aochanarrays"=w192:refnum<k21>[])
            n101 = call "prepDO_focusalign.vi"("rate"=w137, "data"=w127, "bufferAO"=w136) -> ("error out"=w187:errorcluster, "task out"=w188:refnum<k21>)
            n102 = call "prepAI_focusalign.vi"("rate"=w137, "bufferAI"=w136, "triggersource"=w193) -> ("error out"=w189:errorcluster, "header"=w179:dbl[], "task out"=w190:refnum<k21>)
            n103 = call-poly <vilib>:"DAQmx Read.vi"("task/channels in"=w186, "number of samples per channel"=w136, "timeout"=10.0, "error in"=w185) -> ("task out"=w134:refnum<k21>, "data"=w126:i16[][], "error out"=w133:errorcluster)  [unwired: 9 in]
            n104 = To Single Precision Float(number=w126) -> (single precision float=w178:sgl[][])
            n105 = Index Array(array=w178, index (row) #1=0 ("index (row)"), index (row) #2=1 ("index (row)")) -> (element #1=w183:sgl[], element #2=w182:sgl[])  [unwired: 2 in]
            n106 = call "Unscaledtoscaled.vi"("Unscaled Data"=w183, "Header Information"=w179) -> ("Array"=w125:sgl[])  [unwired: 1 in]
            n107 = call "Unscaledtoscaled.vi"("Unscaled Data"=w182, "Header Information"=w179) -> ("Array"=w124:sgl[])  [unwired: 1 in]
            n108 = script code="data=reshape(datain,[bin length(datain)./bin]);\ndataout=mean(data,1);\ndata2=reshape(datain2,[bin length(datain2)./bin]);\ndataout2=mean(data2,1);"("bin"="bin", "datain"=w125, "datain2"=w124) -> ("dataout"=w122:dbl[], "dataout2"=w123:dbl[])  [unwired: 1 in, 1 out]
            n109 = Array Size(array=w122) -> (size(s)=w184:i32)
            n110 = Array Size(array=w123) -> (size(s)=w152:i32)
            n111 = Divide(x=w184, y=w117) -> (x/y=w177:dbl)
            n112 = Divide(x=w152, y=w120) -> (x/y=w121:dbl)
            n113 = Round To Nearest(number=w177) -> (nearest integer value=w116:dbl)
            n114 = Reshape Array(w122, w117, w116) -> (w144:dbl[][])
            n115 = Divide(x=w116, y=3.0) -> (x/y=w108:dbl)
            n116 = Round To Nearest(number=w121) -> (nearest integer value=w118:dbl)
            n117 = Divide(x=w118, y=3.0) -> (x/y=w112:dbl)
            n118 = Multiply(x=w112, y=2.0) -> (x*y=w111:dbl)
            n119 = Multiply(x=w108, y=2.0) -> (x*y=w107:dbl)
            n120 = Array Subset(array=w144, index (row)=0 ("index"), length (row)=6 ("length"), index (col)=w108, length (col)=w107) -> (w141:dbl[][])
            n121 = Reshape Array(w123, w120, w118) -> (w119:dbl[][])
            n122 = Array Subset(array=w119, index (row)=0 ("index"), length (row)=6 ("length"), index (col)=w112, length (col)=w111) -> (w115:dbl[][])
            n123 = Index Array(array=w141, index (row)=0) -> (element=w174:dbl[])  [unwired: 1 in]
            n124 = Index Array(array=w141, index (row)=3) -> (element=w173:dbl[])  [unwired: 1 in]
            n125 = Index Array(array=w141, index (row)=1) -> (element=w171:dbl[])  [unwired: 1 in]
            n126 = Index Array(array=w141, index (row)=4) -> (element=w172:dbl[])  [unwired: 1 in]
            n127 = Index Array(array=w141, index (row)=2) -> (element=w166:dbl[])  [unwired: 1 in]
            n128 = Index Array(array=w141, index (row)=5) -> (element=w165:dbl[])  [unwired: 1 in]
            n129 = Index Array(array=w115, index (row)=0) -> (element=w155:dbl[])  [unwired: 1 in]
            n130 = Index Array(array=w115, index (row)=3) -> (element=w156:dbl[])  [unwired: 1 in]
            n131 = Index Array(array=w115, index (row)=1) -> (element=w158:dbl[])  [unwired: 1 in]
            n132 = Index Array(array=w115, index (row)=4) -> (element=w157:dbl[])  [unwired: 1 in]
            n133 = Index Array(array=w115, index (row)=2) -> (element=w163:dbl[])  [unwired: 1 in]
            n134 = Index Array(array=w115, index (row)=5) -> (element=w164:dbl[])  [unwired: 1 in]
            n135 = Build Array(w174, w173) -> (→"Waveform Graph":dbl[][])
            n136 = Build Array(w171, w172) -> (→"Waveform Graph 2":dbl[][])
            n137 = Build Array(w166, w165) -> (→"Waveform Graph 3":dbl[][])
            n138 = Build Array(w155, w156) -> (→"Waveform Graph 4":dbl[][])
            n139 = Build Array(w158, w157) -> (→"Waveform Graph 5":dbl[][])
            n140 = Build Array(w163, w164) -> (→"Waveform Graph 6":dbl[][])
          }
          frame #3 {
            n141 = flat-sequence {
              tunnel: w258 -> [w266]
              tunnel: w257 -> [w265]
              frame #0 {
                n142 = for {
                  tunnel: w266 -> [w268] mode=indexing
                  tunnel: w265 -> [w267] mode=indexing
                  n143 = call <vilib>:"DAQmx Stop Task.vi"("task/channels in"=w268, "error in"=w267) -> ("task out"=w270:refnum<k21>, "error out"=w269:errorcluster)  [unwired: 12 in]
                  n144 = call <vilib>:"DAQmx Clear Task.vi"("task in"=w270, "error in"=w269) -> ()  [unwired: 13 in, 1 out]
                }
              }
              frame #1 {
                n145 = call "configuration.vi"("command"="get") -> ("config out"=w277:T3)  [unwired: 2 in, 1 out]
                n146 = Unbundle By Name(w277) -> ("Device 1 sampleclock out"=w274:tag, "Device 1 Starttrigger out"=w273:tag)
                n147 = call <vilib>:"DAQmx Disconnect Terminals.vi"("source terminal"=tag "/Dev1/ao/SampleClock", "destination terminal"=w274) -> ("error out"=w271:errorcluster)  [unwired: 13 in]
                n148 = call <vilib>:"DAQmx Disconnect Terminals.vi"("source terminal"=tag "/Dev1/ao/StartTrigger", "destination terminal"=w273, "error in"=w271) -> ()  [unwired: 12 in, 1 out]
              }
            }
            n149 = call <vilib>:"DAQmx Stop Task.vi"("task/channels in"=w256, "error in"=w255) -> ("task out"=w263:refnum<k21>, "error out"=w264:errorcluster)  [unwired: 12 in]
            n150 = call <vilib>:"DAQmx Stop Task.vi"("task/channels in"=w260, "error in"=w259) -> ("task out"=w262:refnum<k21>, "error out"=w261:errorcluster)  [unwired: 12 in]
            n151 = call <vilib>:"DAQmx Clear Task.vi"("task in"=w263, "error in"=w264) -> ()  [unwired: 13 in, 1 out]
            n152 = call <vilib>:"DAQmx Clear Task.vi"("task in"=w262, "error in"=w261) -> ()  [unwired: 13 in, 1 out]
          }
        }
        n153 = Wait (ms)(milliseconds to wait=u32 50) -> ()  [unwired: 1 out]
        n154 = local read "stop"() -> (w14:bool)
      }
      n155 = while {
        stop <- "stop" stop-if-true
        n156 = Boolean To (0,1)(Boolean="y-") -> (0, 1=w295:i16)
        n157 = Boolean To (0,1)(Boolean="y+") -> (0, 1=w294:i16)
        n158 = Boolean To (0,1)(Boolean="x+") -> (0, 1=w297:i16)
        n159 = Boolean To (0,1)(Boolean="x-") -> (0, 1=w296:i16)
        n160 = Negate(x=w295) -> (-x=w289:i16)
        n161 = Negate(x=w296) -> (-x=w288:i16)
        n162 = Add(x=w289, y=w294) -> (x+y=w285:i16)
        n163 = Add(x=w297, y=w288) -> (x+y=w279:i16)
        n164 = local read "ysteps"() -> (w286:i16)
        n165 = Add(x=w286, y=w285) -> (x+y=→"ysteps":i16)
        n166 = local read "xsteps"() -> (w280:i16)
        n167 = Boolean To (0,1)(Boolean="z+") -> (0, 1=w293:i16)
        n168 = Boolean To (0,1)(Boolean="z-") -> (0, 1=w292:i16)
        n169 = Negate(x=w292) -> (-x=w290:i16)
        n170 = local read "zsteps"() -> (w283:i16)
        n171 = Add(x=w293, y=w290) -> (x+y=w282:i16)
        n172 = Add(x=w280, y=w279) -> (x+y=→"xsteps":i16)
        n173 = Add(x=w283, y=w282) -> (x+y=→"zsteps":i16)
        n174 = Wait (ms)(milliseconds to wait=u32 50) -> ()  [unwired: 1 out]
      }
    }
    frame #2 {
      n175 = call "configuration.vi"("command"="get") -> ("config out"=w308:T3)  [unwired: 2 in, 1 out]
      n176 = Unbundle By Name(w308) -> ("AOlines"=w307:tag[], "voltage to Zpos"=w305:i32)
      n177 = Index Array(array=w307, index=w305) -> (element=w306:tag)
      n178 = call <vilib>:"DAQmx Create Task.vi"("new task name"="setpos", "auto cleanup"=TRUE) -> ("task out"=w314:refnum<k21>, "error out"=w312:errorcluster)  [unwired: 12 in]
      n179 = call-poly <vilib>:"DAQmx Create Virtual Channel.vi"("task in"=w314, "physical channels"=w306, "error in"=w312) -> ("task out"=w315:refnum<k21>, "error out"=w311:errorcluster)  [unwired: 11 in]
      n180 = local read "zc"() -> (w304:dbl)
      "finalz" <- w304
      n181 = call-poly <vilib>:"DAQmx Write.vi"("task/channels in"=w315, "data"=w304, "error in"=w311) -> ("task out"=w316:refnum<k21>, "error out"=w317:errorcluster)  [unwired: 10 in, 1 out]
      n182 = call <vilib>:"DAQmx Clear Task.vi"("task in"=w316, "error in"=w317) -> ()  [unwired: 14 out]
    }
  }
